vi "labview2.vi"(11 "km/h":dbl) -> (3 "ms/s":dbl)   [LabVIEW 2015]
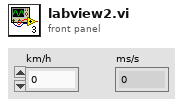
[diagram p1: front panel]
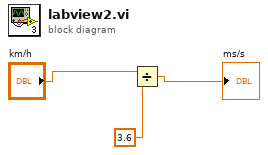
[diagram p0: block diagram]
diagram:
  n1 = Divide(x="km/h", y=3.6) -> (x/y=→"ms/s":dbl)
